vi "TLCCS Get Scan Data.vi"(8 "error in (no error)":errorcluster {"code" format="%.0x"}, 11 "instrument handle":refnum<visa-resource-name>) -> (0 "error out":errorcluster {"code" format="%.0x"}, 2 "Data":dbl[](array[numeric]) format="%.2p", 3 "instrument handle out":refnum<visa-resource-name>)   [LabVIEW 2020]
doc: "This VI reads out the processed scan data.\n\nNote:\nWhen the raw scan data is overexposed, so that a proper data processing is not possible, the VI returns\n\nVI_ERROR_SCAN_DATA_INVALID (-1074001917) \n\nand all data points are set to zero (0.0)."
uses:
  tlccs_32.dll
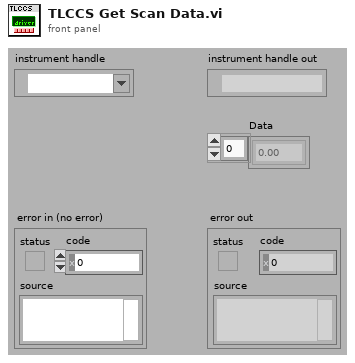
[diagram p1: front panel]
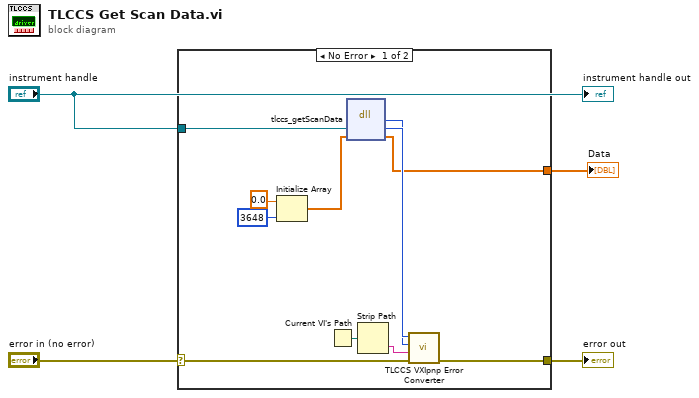
[diagram p0: block diagram]
diagram:
  n1 = case shown="No Error" "error in (no error)" {
    selector: "error in (no error)" -> [w10 w16]
    tunnel: [w9 w16] -> w4
    tunnel: "instrument handle" -> [w14 _]
    tunnel: [w5 _] -> w1
    frame No Error {
      n2 = Initialize Array(0.0 ("element"), 3648 ("dimension size")) -> (w8:dbl[])
      n3 = Current VI's Path() -> (path=w15:path)
      n4 = dll-call lib="tlccs_32.*" fn="tlccs_getScanData"("Instrument Handle"=w14, "Data"=w8) -> (w12:i32, "Instrument Handle"=w13:u32, "Data"=w5:dbl[])  [unwired: 3 in, 2 out]
      n5 = Strip Path(path=w15) -> (name=w11:string)  [unwired: 1 out]
      n6 = call "TLCCS VXIpnp Error Converter.vi"("error in (no error)"=w10, "name of VI (\"\")"=w11, "CVI error code (0)"=w12, "instrument handle"=w13) -> ("error out"=w9:errorcluster)  [unwired: 6 in, 1 out]
    }
    frame Error {
    }
  }
  "error out" <- w4
  "Data" <- w1
  "instrument handle out" <- "instrument handle"
